vi "Read Number Variable.vi"(2 "error in (no error)":errorcluster, 3 "Name":string) -> (0 "error out":errorcluster, 1 "number":dbl)   [LabVIEW 2014]
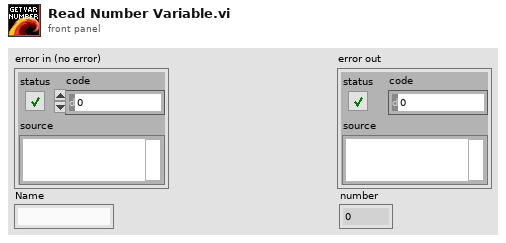
[diagram p1: front panel]
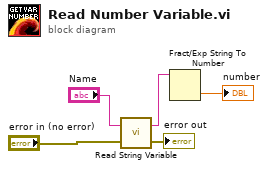
[diagram p0: block diagram]
diagram:
  n1 = call "Read String Variable.vi"("error in (no error)"="error in (no error)", "Name"="Name") -> ("error out"=→"error out":errorcluster, "Variable"=w2:string)
  n2 = Fract/Exp String To Number(string=w2) -> (number=→"number":dbl)  [unwired: 3 in, 1 out]
